vi "Send Subscription List To Robot.vi"(8 "error in (no error)":errorcluster, 10 "Selected parameters 2":refnum<vi>, 11 "Inventory":T1) -> (0 "error out":errorcluster)   [LabVIEW 2016]
uses:
  inventory type def.ctl
  subscription type def.ctl
  Communication Global variables.vi
  <vilib>/addons/_JKI.lib/REST Client/classes/REST Client/REST Client.lvclass
  <vilib>/addons/_JKI.lib/Serialization/JSON/JKI JSON Serialization.lvlib
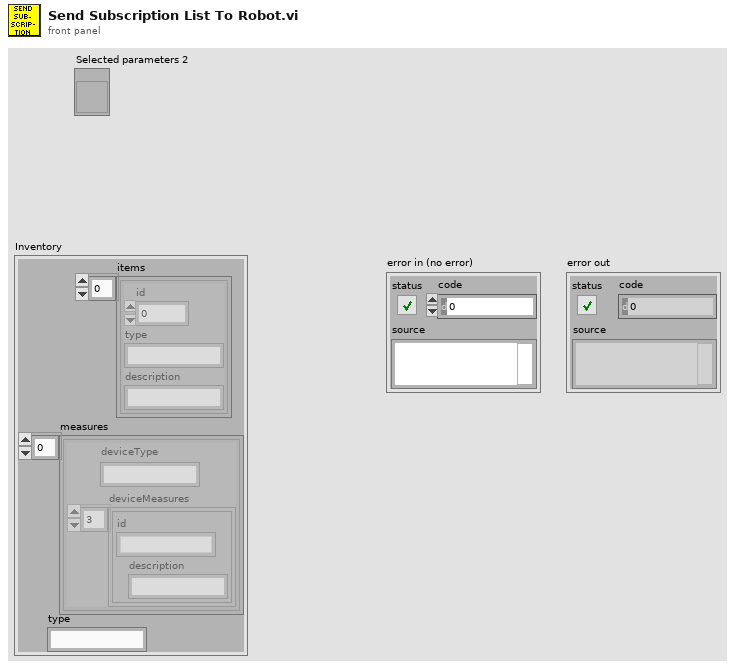
[diagram p1: front panel]
types:
  T1 = typedef "inventory type def.ctl" = cluster{"items":cluster{"id":u8, "type":string, "description":string}[], "measures":cluster{"deviceType":string, "deviceMeasures":cluster{"id":string, "description":string}[]}[], "type":string}
  T2 = cluster{"id":u8, "type":string, "description":string}[]
  T3 = cluster{"deviceType":string, "deviceMeasures":cluster{"id":string, "description":string}[]}[]
  T4 = typedef "subscription type def.ctl" = cluster{"type":string, "subscription":cluster{"itemId":i32, "measurementId":string}[]}
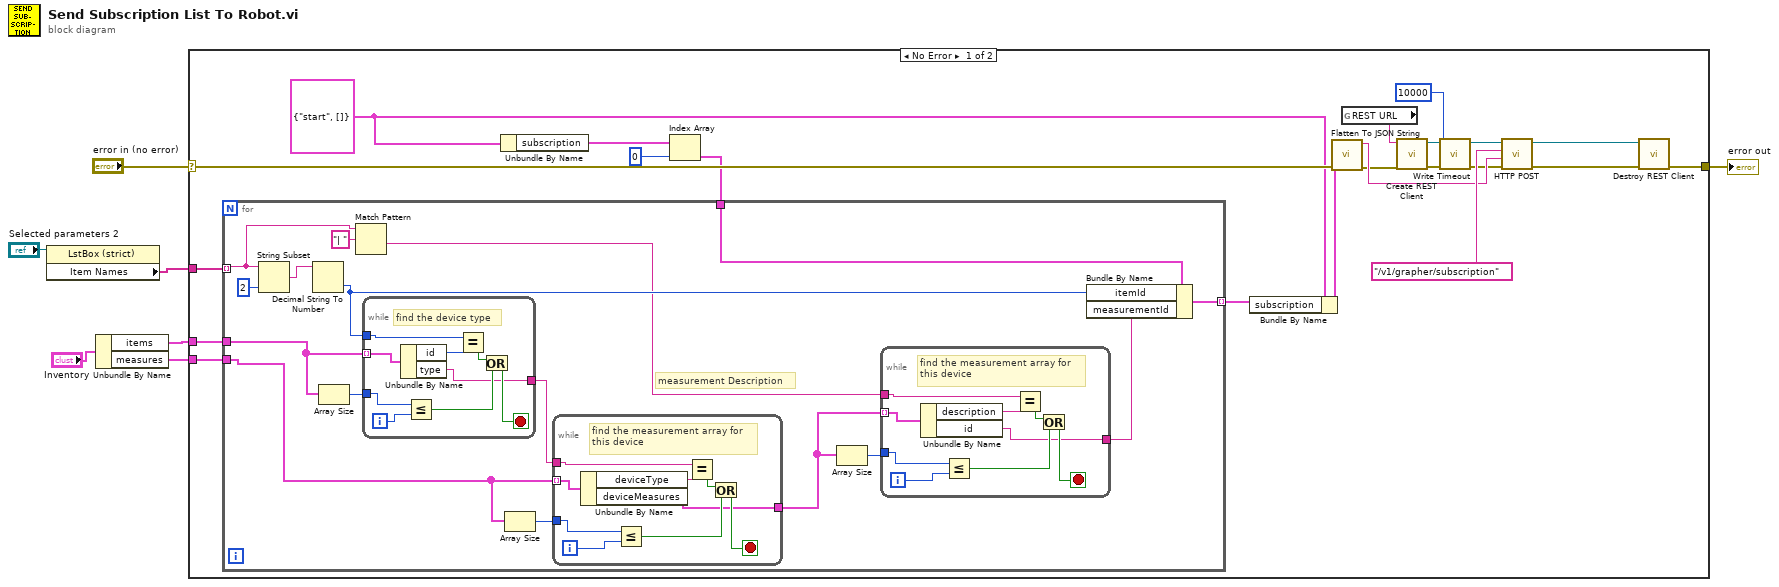
[diagram p0: block diagram]
diagram:
  n1 = property class="LstBox (strict)"(reference="Selected parameters 2") -> ("Item Names"=w4:string[])  [unwired: 1 in, 2 out]
  n2 = Unbundle By Name("Inventory") -> ("items"=w1:T2, "measures"=w2:T3)
  n3 = case shown="No Error" "error in (no error)" {
    selector: "error in (no error)" -> [w23 w73]
    tunnel: [w24 w73] -> w6
    tunnel: w4 -> [w19 _]
    tunnel: w2 -> [w9 _]
    tunnel: w1 -> [w8 _]
    frame No Error {
      w18 = T4 {"type"="start", "subscription"=[]} ("Subscription list")
      n4 = Unbundle By Name(w18) -> ("subscription"=w17:cluster{"itemId":i32, "measurementId":string}[])
      n5 = Index Array(array=w17, index=0) -> (element=w15:cluster{"itemId":i32, "measurementId":string})
      n6 = for {
        tunnel: w19 -> [w34] mode=indexing
        tunnel: [w43] -> w21 mode=indexing
        tunnel: w15 -> [w42]
        tunnel: w9 -> [w36]
        tunnel: w8 -> [w40]
        # "measurement Description"
        n7 = String Subset(string=w34, length (rest)=2 ("length (rest)")) -> (substring=w44:string)  [unwired: 1 in]
        n8 = Decimal String To Number(string=w44) -> (number=w41:i32)  [unwired: 2 in, 1 out]
        n9 = Array Size(array=w40) -> (size(s)=w39:i32)
        n10 = Match Pattern(string=w34, regular expression="| ") -> (after substring=w33:string)  [unwired: 1 in, 3 out]
        n11 = while {
          tunnel: w41 -> [w72]
          tunnel: w40 -> [w71] mode=indexing
          tunnel: w39 -> [w67]
          tunnel: [w64] -> w38
          i -> [w68]
          stop <- w65 stop-if-true
          # "find the device type"
          n12 = Unbundle By Name(w71) -> ("id"=w70:u8, "type"=w64:string)
          n13 = Less Or Equal?(x=w67, y=w68) -> (x <= y?=w66:bool)
          n14 = Equal?(x=w72, y=w70) -> (x = y?=w69:bool)
          n15 = Or(x=w69, y=w66) -> (x .or. y?=w65:bool)
        }
        n16 = Array Size(array=w36) -> (size(s)=w37:i32)
        n17 = while {
          tunnel: w38 -> [w63]
          tunnel: w36 -> [w62] mode=indexing
          tunnel: w37 -> [w58]
          tunnel: [w55] -> w31
          i -> [w59]
          stop <- w56 stop-if-true
          # "find the measurement array for\nthis device"
          n18 = Unbundle By Name(w62) -> ("deviceType"=w61:string, "deviceMeasures"=w55:cluster{"id":string, "description":string}[])
          n19 = Less Or Equal?(x=w58, y=w59) -> (x <= y?=w57:bool)
          n20 = Equal?(x=w63, y=w61) -> (x = y?=w60:bool)
          n21 = Or(x=w60, y=w57) -> (x .or. y?=w56:bool)
        }
        n22 = Array Size(array=w31) -> (size(s)=w32:i32)
        n23 = while {
          tunnel: w33 -> [w54]
          tunnel: w31 -> [w53] mode=indexing
          tunnel: w32 -> [w49]
          tunnel: [w46] -> w30
          i -> [w50]
          stop <- w47 stop-if-true
          # "find the measurement array for\nthis device"
          n24 = Unbundle By Name(w53) -> ("description"=w52:string, "id"=w46:string)
          n25 = Less Or Equal?(x=w49, y=w50) -> (x <= y?=w48:bool)
          n26 = Equal?(x=w54, y=w52) -> (x = y?=w51:bool)
          n27 = Or(x=w51, y=w48) -> (x .or. y?=w47:bool)
        }
        n28 = Bundle By Name(cluster=w42, "itemId"=w41, "measurementId"=w30) -> (w43:cluster{"itemId":i32, "measurementId":string})
      }
      n29 = Bundle By Name(cluster=w18, "subscription"=w21) -> (w20:T4)
      n30 = call <vilib>:"Flatten To JSON String.vi"("error in (no error)"=w23, "Variant"=w20) -> ("error out"=w22:errorcluster, "JSON String"=w26:string)  [unwired: 8 in]
      n31 = global read "Communication Global variables.vi" "REST URL"() -> (w27:string)
      n32 = call <vilib>:"Create REST Client.vi"("error in (no error)"=w22, "Base URL"=w27) -> ("error out"=w12:errorcluster, "REST Client out"=w14:refnum<class "REST Client.lvclass">)  [unwired: 8 in]
      n33 = call-dynamic "Write Timeout.vi"("error in (no error)"=w12, "Timeout"=10000, "REST Client in"=w14) -> ("error out"=w11:errorcluster, "REST Client out"=w13:refnum<class "REST Client.lvclass">)  [unwired: 7 in]
      n34 = call-dynamic "HTTP POST.vi"("error in (no error)"=w11, "Request body"=w26, "Path"="/v1/grapher/subscription", "REST Client in"=w13) -> ("error out"=w25:errorcluster, "REST Client out"=w28:refnum<class "REST Client.lvclass">)  [unwired: 2 in, 4 out]
      n35 = call-dynamic "Destroy REST Client.vi"("error in (no error)"=w25, "REST Client in"=w28) -> ("error out"=w24:errorcluster)  [unwired: 9 in]
    }
    frame Error {
    }
  }
  "error out" <- w6
